vi "AutoFollowRelativeTrajectoryAndRevShoot.vi"(8 "error in (no error)":errorcluster, 9 "TimeOut (s)":dbl, 10 "End Orientation":dbl, 11 "Trajectory":T1 {"States"."POSE"."ROTATION"."SIN" format="%13.4f"; "States"."POSE"."ROTATION"."COS" format="%13.4f"; "States"."POSE"."ROTATION"."VALUE" format="%13.4f"; "States"."POSE"."TRANSLATION"."Y" format="%14.3f"; "States"."POSE"."TRANSLATION"."X" format="%14.3f"; "TotalTImeSecs" format="%20.3f"}) -> (0 "error out":errorcluster)   [LabVIEW 2023]
doc: "Wrapper class for drive straight"
uses:
  <vilib>/Rock Robotics/WPI/ThirdParty/JAS_Junk/TrajLib/TypeDef/TRAJECTORY.ctl
  <vilib>/Rock Robotics/WPI/ThirdParty/JAS_Junk/TrajLib/TypeDef/TRAJ_STATE.ctl
  <vilib>/Rock Robotics/WPI/ThirdParty/JAS_Junk/TrajLib/TypeDef/POSE2D.ctl
  <vilib>/Rock Robotics/WPI/ThirdParty/JAS_Junk/TrajLib/TypeDef/TRANSLATION2D.ctl
  <vilib>/Rock Robotics/WPI/ThirdParty/JAS_Junk/TrajLib/TypeDef/ROTATION2D.ctl
  <vilib>/Utility/semaphor.llb/Obtain Semaphore Reference.vi
  <vilib>/Rock Robotics/WPI/ThirdParty/JAS_Junk/TrajLib/Timer_Reset.vi
  <vilib>/Rock Robotics/WPI/ThirdParty/JAS_Junk/TrajLib/Trajectory_Library.lvlib
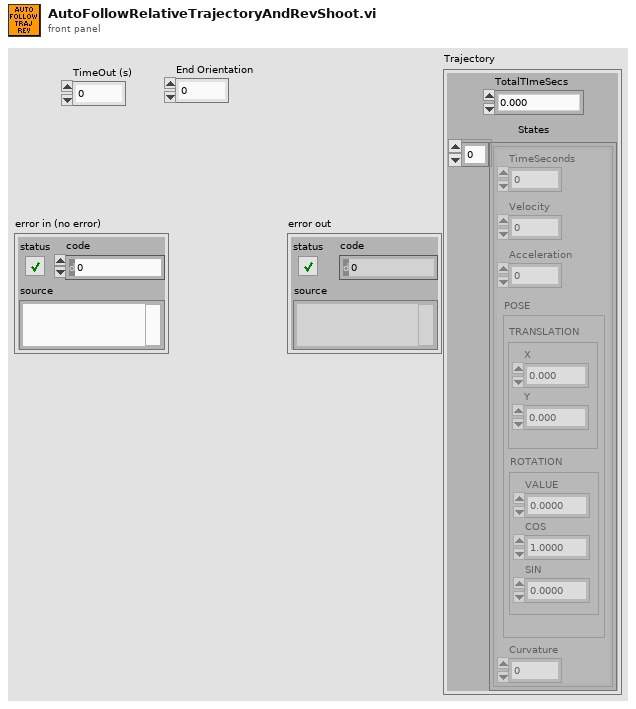
[diagram p1: front panel]
types:
  T1 = typedef "Trajectory_Library.lvlib/TRAJECTORY.ctl" = cluster{"TotalTImeSecs":dbl, "States":T2[]}
  T2 = typedef "Trajectory_Library.lvlib/TRAJ_STATE.ctl" = cluster{"TimeSeconds":dbl, "Velocity":dbl, "Acceleration":dbl, "POSE":T3, "Curvature":dbl}
  T3 = typedef "Trajectory_Library.lvlib/POSE2D.ctl" = cluster{"TRANSLATION":T4, "ROTATION":T5}
  T4 = typedef "Trajectory_Library.lvlib/TRANSLATION2D.ctl" = cluster{"X":dbl, "Y":dbl}
  T5 = typedef "Trajectory_Library.lvlib/ROTATION2D.ctl" = cluster{"VALUE":dbl, "COS":dbl, "SIN":dbl}
  T6 = typedef "Trajectory_Library.lvlib/TIMER.ctl" = cluster{"StartTime":dbl, "Accumulated TIme":dbl, "Running":bool, "semaphore":T7}
  T7 = typedef "Semaphore RefNum" = refnum<k1>
  T8 = typedef "Trajectory_Library.lvlib/CHASSIS_SPEEDS.ctl" = cluster{"vX":dbl, "vY":dbl, "vOmega":dbl}
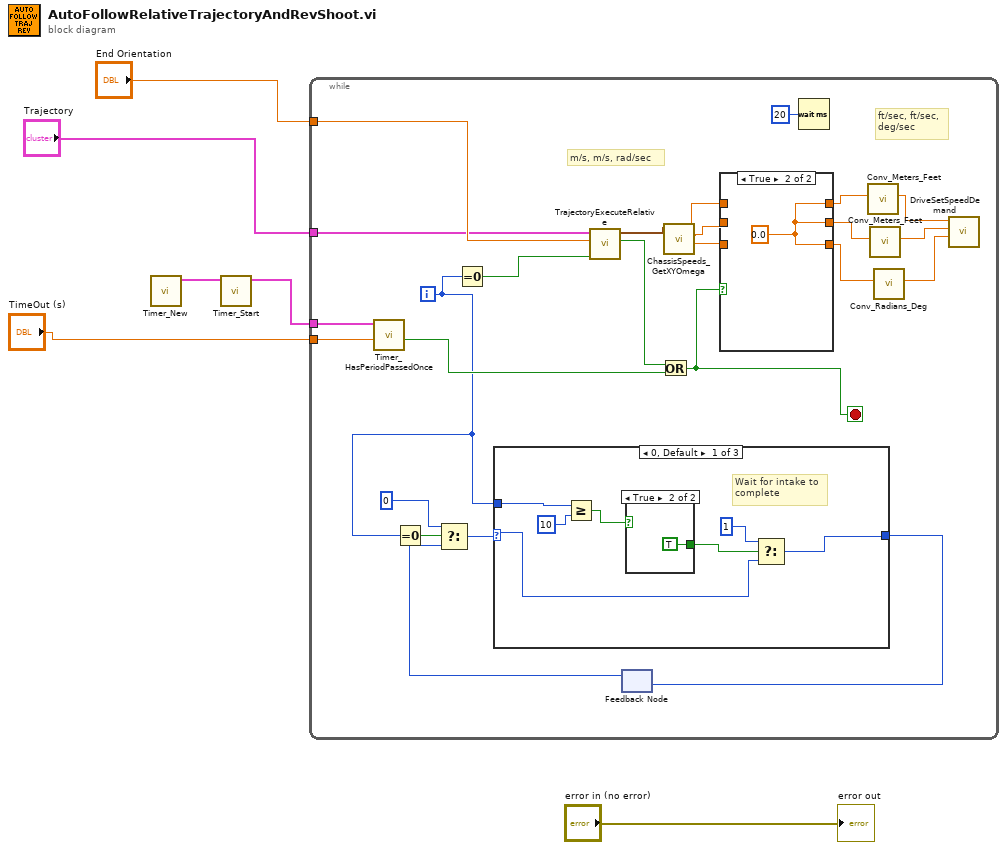
[diagram p0: block diagram]
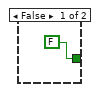
[diagram p2: hidden frame]
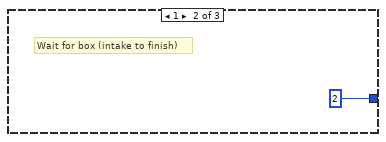
[diagram p3: hidden frame]
diagram:
  n1 = call <vilib>:"Timer_New.vi"() -> ("TIMER"=w5:T6)  [unwired: 11 in]
  n2 = call <vilib>:"Timer_Start.vi"("in Timer"=w5) -> ("out Timer"=w4:T6)  [unwired: 10 in]
  n3 = while {
    tunnel: w4 -> [w31]
    tunnel: "TimeOut (s)" -> [w30]
    tunnel: "Trajectory" -> [w26]
    tunnel: "End Orientation" -> [w27]
    i -> [w7]
    stop <- w13 stop-if-true
    # "ft/sec, ft/sec,\ndeg/sec"
    # "m/s, m/s, rad/sec"
    n4 = call <vilib>:"Timer_HasPeriodPassedOnce.vi"("Period"=w30, "in Timer"=w31) -> ("Expired"=w29:bool)  [unwired: 7 in, 2 out]
    n5 = Equal To 0?(x=w7) -> (x = 0?=w12:bool)
    n6 = Equal To 0?(x=w7) -> (x = 0?=w25:bool)
    n7 = call "TrajectoryExecuteRelative.vi"("Init"=w25, "End Relative\nOrientation Deg"=w27, "Trajectory"=w26) -> ("Done"=w24:bool, "Chassis Velocity Target Met,Met,Rad"=w20:T8)  [unwired: 6 in, 1 out]
    n8 = feedback #1() -> (w8:i32)  [unwired: 1 in]
    n9 = Select(t=0, s=w12, f=w8) -> (s? t:f=w10:i32)
    n10 = case shown="0, Default" w10 {
      selector: w10 -> [w34 _ w42]
      tunnel: [w32 2 ("t") w42] -> w9
      tunnel: w7 -> [w36 _ _]
      frame 0, Default {
        # "Wait for intake to\ncomplete"
        n11 = Greater Or Equal?(x=w36, y=10) -> (x >= y?=w38:bool)
        n12 = case shown="True" w38 {
          tunnel: [FALSE TRUE] -> w35
          frame False {
          }
          frame True {
          }
        }
        n13 = Select(t=1, s=w35, f=w34) -> (s? t:f=w32:i32)
      }
      frame 1 {
        # "Wait for box (intake to finish)"
      }
      frame 2 {
      }
    }
    n14 = feedback-in #1(w9) -> ()
    n15 = Or(x=w24, y=w29) -> (x .or. y?=w13:bool)
    n16 = call <vilib>:"ChassisSpeeds_GetXYOmega.vi"("CHASSIS"=w20) -> ("vAngular"=w23:dbl, "vY"=w22:dbl, "vX"=w21:dbl)  [unwired: 8 in]
    n17 = case shown="True" w13 {
      tunnel: w21 -> [w45 _]
      tunnel: w22 -> [w44 _]
      tunnel: w23 -> [w43 _]
      tunnel: [w45 w46] -> w19
      tunnel: [w44 w46] -> w17
      tunnel: [w43 w46] -> w15
      frame False {
      }
      frame True {
        w46 = 0.0 ("XSpeedDemand")
      }
    }
    n18 = Wait (ms)(milliseconds to wait=u32 20) -> ()  [unwired: 1 out]
    n19 = call <vilib>:"Conv_Meters_Feet.vi"("Meters"=w19) -> ("Feet"=w18:dbl)  [unwired: 10 in]
    n20 = call <vilib>:"Conv_Meters_Feet.vi"("Meters"=w17) -> ("Feet"=w16:dbl)  [unwired: 10 in]
    n21 = call <vilib>:"Conv_Radians_Deg.vi"("Radians"=w15) -> ("Degrees"=w14:dbl)  [unwired: 10 in]
    n22 = call "DriveSetSpeedDemand.vi"("ASpeedDemand (d/s)"=w14, "YSpeedDemand (ft/s)"=w16, "XSpeedDemand (ft/s)"=w18) -> ()  [unwired: 9 in]
  }
  "error out" <- "error in (no error)"
